vi "Apply delay.vi"(0 "reference in":refnum<class "Force Curve_tdms.lvclass">, 5 "error in (no error)":errorcluster) -> (14 "reference out":refnum<class "Force Curve_tdms.lvclass">, 16 "# of samples":dbl, 19 "error out":errorcluster)   [LabVIEW 2019, in "Force Curve_tdms.lvclass"]
doc: "This takes to account the delay time of the slowest time constant of the afm control system"
uses:
  Force Curve_tdms.lvclass
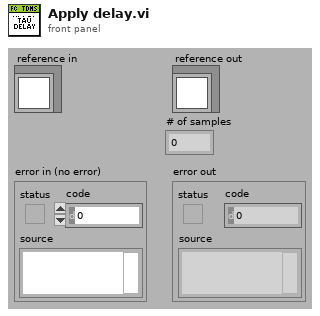
[diagram p1: front panel]
types:
  T1 = typedef "Force Curve_tdms.lvclass/ObjectAttributes.ctl" = cluster{"MyAttribute":dbl, "Processed data":waveform(dbl)[], "Fcurve Raw Metadata":T2, "Fcurve Metadata":T3, "Fcurve index":T4, "Tau Delay (ms)":dbl, "Contact Spread of dev":dbl, "Fcurve":T5}
  T2 = typedef "TDMS_DataHandler.lvclass/Fcurve Meta data.ctl" = cluster{"property names":string[], "property values":variant[]}
  T3 = typedef "Force Curve_tdms.lvclass/Fcurve Meta data analysis.ctl" = cluster{"dt (us)":dbl, "Dec Factor":dbl, "Z piezo Sensitivity (nm/V)":dbl, "K (N/m)":dbl, "Sp (V)":dbl, "Contact (ms)":dbl, "Zpos contact":dbl, "Vel_app (nm/s)":dbl, "Vel_ret (nm/s)":dbl, "deltaV (nm)":dbl, "Def_V0 (v)":dbl, "Decimating Factor":dbl}
  T4 = typedef "Force Curve_tdms.lvclass/Fcurve Index .ctl" = cluster{"Setpoint index":i32, "Max force index":i32, "Contact point index":i32, "Appoach indices":cluster{"Start":i32, "End":i32}, "Contact indices":cluster{"Start":i32, "End":i32}, "Retract indices":cluster{"Start":i32, "End":i32}}
  T5 = typedef "Force Curve_tdms.lvclass/Force Curve data.ctl" = cluster{"Approach":cluster{"X":dbl[], "Y":dbl[]}, "Contact":cluster{"X":dbl[], "Y":dbl[]}, "Retract":cluster{"X":dbl[], "Y":dbl[]}}
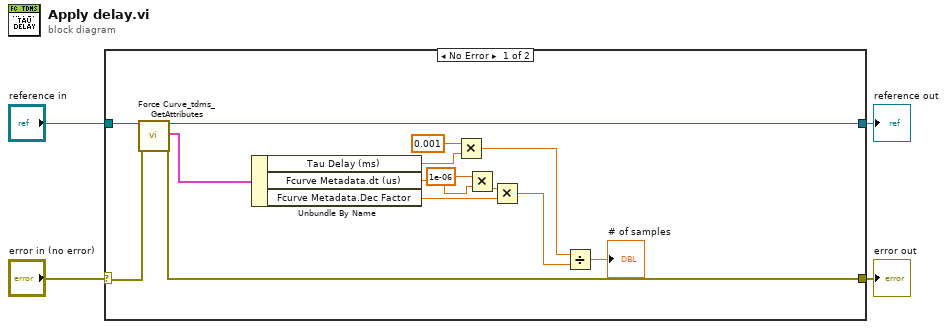
[diagram p0: block diagram]
diagram:
  n1 = case shown="No Error" "error in (no error)" {
    selector: "error in (no error)" -> [w16 w20]
    tunnel: [w15 w20] -> w3
    tunnel: [w17 w19] -> w1
    tunnel: "reference in" -> [w18 w19]
    frame No Error {
      n2 = call "Force Curve_tdms_GetAttributes.vi"("reference in"=w18, "error in (no error)"=w16) -> ("reference out"=w17:refnum<class "Force Curve_tdms.lvclass">, "attributes"=w14:T1, "error out"=w15:errorcluster)  [unwired: 14 in, 1 out]
      n3 = Unbundle By Name(w14) -> ("Tau Delay (ms)"=w11:dbl, "Fcurve Metadata.dt (us)"=w7:dbl, "Fcurve Metadata.Dec Factor"=w13:dbl)
      n4 = Multiply(x=0.001, y=w11) -> (x*y=w9:dbl)
      n5 = Multiply(x=1e-06, y=w7) -> (x*y=w5:dbl)
      n6 = Multiply(x=w5, y=w13) -> (x*y=w12:dbl)
      n7 = Divide(x=w9, y=w12) -> (x/y=→"# of samples":dbl)
    }
    frame Error {
    }
  }
  "error out" <- w3
  "reference out" <- w1
